vi "uA_change_lable_unit.vi"(11 "Range - Shunts":T1) -> (3 "unit":string)   [LabVIEW 2015]
uses:
  Range_Shunt_selector.ctl
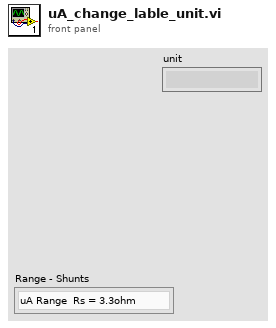
[diagram p1: front panel]
types:
  T1 = typedef "Range_Shunt_selector.ctl" = enum16{"uA Range  Rs = 3.3ohm", "mA Range Rs = 3.3Ohm", "mA Range Rs = 1Ohm", "mA Range Rs = 1Ohm - X2"}
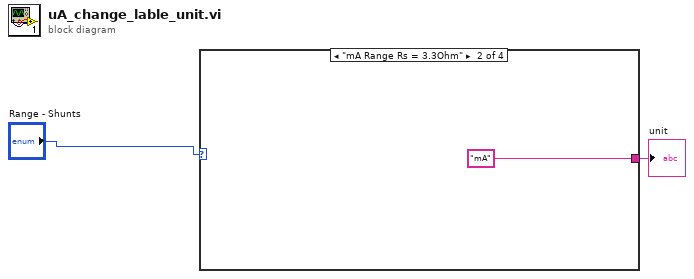
[diagram p0: block diagram]
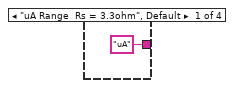
[diagram p2: hidden frame]
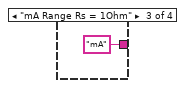
[diagram p3: hidden frame]
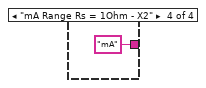
[diagram p4: hidden frame]
diagram:
  n1 = case shown="\"mA Range Rs = 3.3Ohm\"" "Range - Shunts" {
    tunnel: ["uA" "mA" "mA" "mA"] -> w1
    frame "uA Range  Rs = 3.3ohm", Default {
    }
    frame "mA Range Rs = 3.3Ohm" {
    }
    frame "mA Range Rs = 1Ohm" {
    }
    frame "mA Range Rs = 1Ohm - X2" {
    }
  }
  "unit" <- w1
